vi "CommunicationFormat_SetHeaderLength.vi"(8 "error in (no error)":errorcluster, 10 "Long Communication Header?":bool, 11 "OXYGEN Ref In":refnum<visa-resource-name>) -> (0 "error out":errorcluster, 1 "communication_data":T1, 3 "OXYGEN Ref Out":refnum<visa-resource-name>)   [LabVIEW 2020, in "OXYGEN_Datastream.lvlib"]
doc: "Sets whether query responses should generate the long or short form of the header.\nParameter Name Type Range Default."
uses:
  OXYGEN_Datastream.lvlib
  TypeDefs/Cluster_RawCommData.ctl
  TypeDefs/Modes_FGV_OutputHeaderFormat.ctl
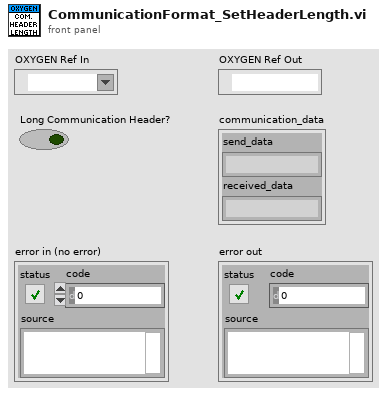
[diagram p1: front panel]
types:
  T1 = typedef "OXYGEN_Datastream.lvlib/Cluster_RawCommData.ctl" = cluster{"send_data":string, "received_data":string}
  T2 = typedef "OXYGEN_Datastream.lvlib/Modes_FGV_OutputHeaderFormat.ctl" = enum16{"Set", "Get"}
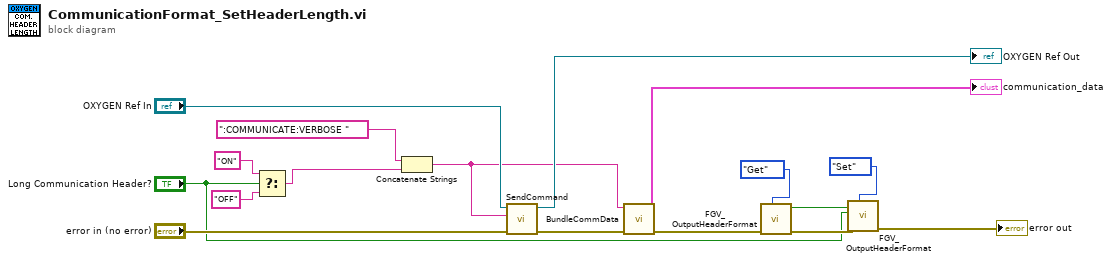
[diagram p0: block diagram]
diagram:
  n1 = Select(t="ON", s="Long Communication Header?", f="OFF") -> (s? t:f=w8:string)
  n2 = Concatenate Strings(":COMMUNICATE:VERBOSE ", w8) -> (w14:string)
  n3 = call "SendCommand.vi"("error in (no error)"="error in (no error)", "String to Send"=w14, "OXY_SCPI Reseource In"="OXYGEN Ref In") -> ("error out"=w13:errorcluster, "OXY_SCPI Reseource Out"=→"OXYGEN Ref Out":refnum<visa-resource-name>)  [unwired: 7 in]
  n4 = call "BundleCommData.vi"("error in (no error)"=w13, "send_data"=w14) -> ("error out"=w4:errorcluster, "communication_data"=→"communication_data":T1)  [unwired: 8 in]
  n5 = call "FGV_OutputHeaderFormat.vi"("Mode"=Modes_FGV_OutputHeaderFormat."Get", "error in (no error)"=w4) -> ("error out"=w5:errorcluster, "Header On?"=w2:bool)  [unwired: 7 in, 1 out]
  n6 = call "FGV_OutputHeaderFormat.vi"("Mode"=Modes_FGV_OutputHeaderFormat."Set", "error in (no error)"=w5, "Long Header?"="Long Communication Header?", "Header On?"=w2) -> ("error out"=→"error out":errorcluster)  [unwired: 5 in, 2 out]
